vi "Billard2023.vi"() -> ()   [LabVIEW 2022 SP3]
doc: "This VI uses computer vision to score a game of french pool.\nSelect the sequence of png images you want to analyse and let the magic happen...\n\nAuthors : Romain Lattion & Ryan Svoboda"
panel:
  out "Running Matlab...":string
  out "percentage":dbl
  out "slide":dbl(slide) scale=0.0..100.0
  in  "Create Matlab scoresheet":bool
  in  "Line type":string(combo)="-*"
  in  "Band touch lose":u32(colorbox)=16711680
  in  "Band touch win":u32(colorbox)=65280
  in  "Select the sequence (folder)":path
  out "?":picture
  # "Romain Lattion & Ryan Svoboda"
  # "Billard 2023"
  # "Loading...       %"
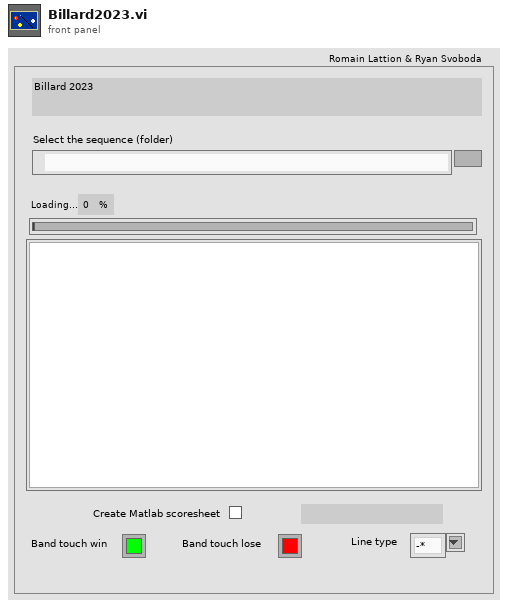
[diagram p1: front panel]
types:
  T1 = typedef "imagedata.ctl" = cluster{"image type":i32, "image depth":i32, "image":u8[], "mask":u8[], "colors":u32[], "Rectangle":cluster{"left":i16, "top":i16, "right":i16, "bottom":i16}}
  T2 = enum16{"open", "replace", "create", "open or create", "replace or create", "replace or create with confirmation"}
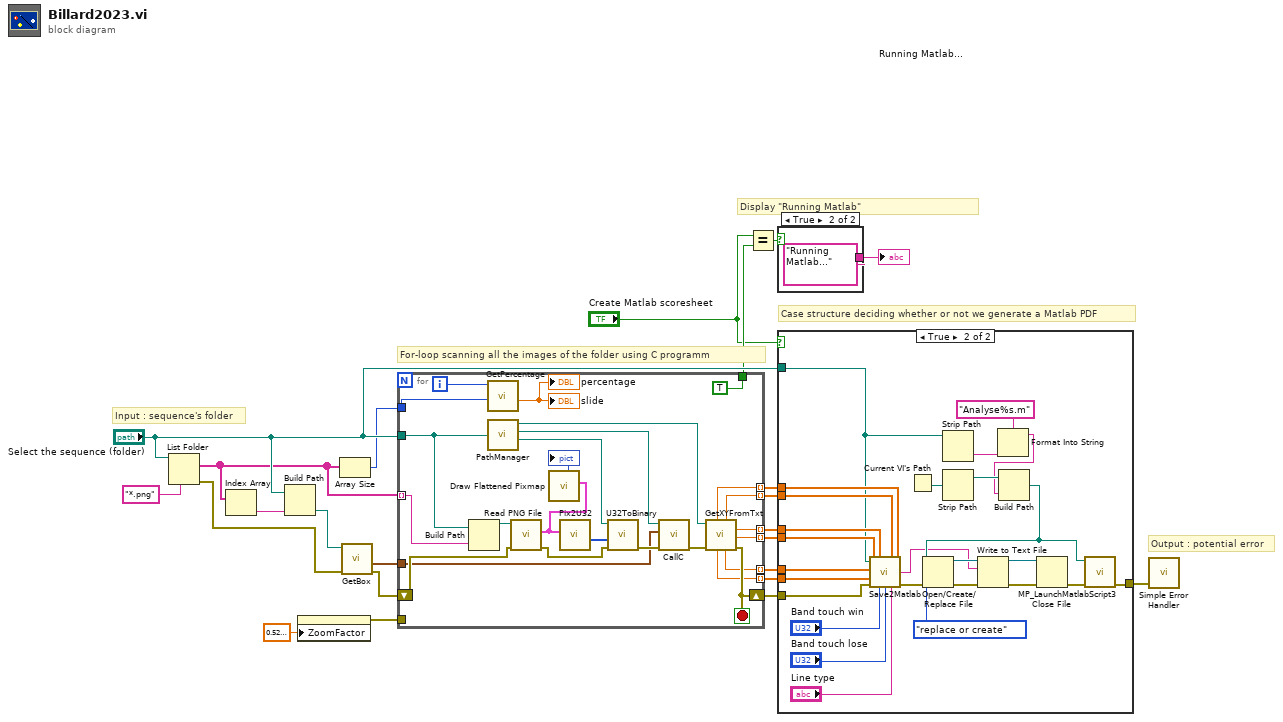
[diagram p0: block diagram]
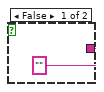
[diagram p2: hidden frame]
diagram:
  # "Output : potential error"
  # "Input : sequence's folder"
  # "Display \"Running Matlab\""
  # "Case structure deciding whether or not we generate a Matlab PDF"
  # "For-loop scanning all the images of the folder using C programm"
  n1 = List Folder(path="Select the sequence (folder)", pattern="*.png") -> (filenames=w12:string[], error out=w17:errorcluster)  [unwired: 2 in, 2 out]
  n2 = Index Array(array=w12) -> (element=w13:string)  [unwired: 1 in]
  n3 = Build Path(base path="Select the sequence (folder)", name or relative path=w13) -> (appended path=w18:path)
  n4 = property class="Pict"("ZoomFactor"=sgl 0.53 ("Zoom Factor")) -> (error out=w22:errorcluster)  [unwired: 2 in, 1 out]
  n5 = Array Size(array=w12) -> (size(s)=w11:i32)
  n6 = call "GetBox.vi"("error in (no error)"=w17, "path to a png image"=w18) -> ("error out"=w16:errorcluster, "edges coordinates"=w15:cluster{u32, u32, u32, u32})  [unwired: 8 in]
  n7 = for {
    tunnel: "Select the sequence (folder)" -> [w25]
    tunnel: w22 -> [_]
    shift-right: [w32] -> w20
    shift-left: w16 -> [w46]
    tunnel: [w26] -> w9 mode=indexing
    tunnel: [w28] -> w8 mode=indexing
    tunnel: [w31] -> w4 mode=indexing
    tunnel: [w30] -> w3 mode=indexing
    tunnel: [w29] -> w2 mode=indexing
    tunnel: [w27] -> w1 mode=indexing
    tunnel: w15 -> [w36]
    tunnel: w12 -> [w42] mode=indexing
    tunnel: w11 -> [w41]
    tunnel: [TRUE] -> w7
    i -> [w39]
    stop <- w32 stop-if-true
    n8 = Build Path(base path=w25, name or relative path=w42) -> (appended path=w48:path)
    n9 = call "GetPercentage.vi"("total number"=w41, "current number"=w39) -> ("percentage"=→"slide" →"percentage":dbl)  [unwired: 9 in]
    n10 = call "PathManager.vi"("path to sequence folder"=w25) -> ("path to Pixmap.bin"=w38:path, "path to Pix2Pos.exe"=w35:path, "path to Pos.txt"=w33:path)  [unwired: 8 in]
    n11 = call <vilib>:"Read PNG File.vi"("error in (no error)"=w46, "path to PNG file"=w48) -> ("error out"=w43:errorcluster, "image data"=w45:T1)  [unwired: 7 in, 1 out]
    n12 = call <vilib>:"Draw Flattened Pixmap.vi"("image data"=w45) -> ("new picture"=→"?":picture)  [unwired: 8 in]
    n13 = call "Pix2U32.vi"("input cluster"=w45) -> ("pixmap"=w44:u32[])  [unwired: 10 in]
    n14 = call "U32ToBinary.vi"("error in"=w43, "pixmap"=w44, "path to pixmap.bin"=w38) -> ("error out"=w37:errorcluster)  [unwired: 8 in]
    n15 = call "CallC.vi"("error in (no error)"=w37, "Edges"=w36, "path to Pix2Pos.exe"=w35) -> ("error out"=w34:errorcluster)  [unwired: 8 in]
    n16 = call "GetXYFromTxt.vi"("error in"=w34, "path to pos.txt"=w33) -> ("error out"=w32:errorcluster, "Yy"=w30:dbl, "Xy"=w31:dbl, "Xw"=w29:dbl, "Yr"=w28:dbl, "Yw"=w27:dbl, "Xr"=w26:dbl)  [unwired: 3 in]
  }
  n17 = Equal?(x="Create Matlab scoresheet", y=w7) -> (x = y?=w5:bool)
  n18 = case shown="True" w5 {
    tunnel: ["" "Running Matlab..."] -> w10
    frame False {
    }
    frame True {
    }
  }
  "Running Matlab..." <- w10
  n19 = case shown="True" "Create Matlab scoresheet" {
    tunnel: w20 -> [w51 w77]
    tunnel: [w51 w76] -> w19
    tunnel: "Select the sequence (folder)" -> [_ w52]
    tunnel: w9 -> [_ w75]
    tunnel: w8 -> [_ w74]
    tunnel: w4 -> [_ w73]
    tunnel: w3 -> [_ w72]
    tunnel: w2 -> [_ w71]
    tunnel: w1 -> [_ w70]
    frame False {
    }
    frame True {
      n20 = call "Save2Matlab.vi"("Xr"=w75, "Yr"=w74, "Line"="Line type", "Band touch loose"="Band touch lose", "Xy"=w73, "Band touch win"="Band touch win", "Yy"=w72, "Path"=w52, "Xw"=w71, "Yw"=w70, "error in (no error)"=w77) -> ("Completed Matlab script"=w53:string, "error out"=w56:errorcluster)  [unwired: 3 in]
      n21 = Current VI's Path() -> (path=w69:path)
      n22 = Strip Path(path=w52) -> (name=w62:string)  [unwired: 1 out]
      n23 = Strip Path(path=w69) -> (stripped path=w68:path)  [unwired: 1 out]
      n24 = Format Into String(format string="Analyse%s.m", w62) -> (resulting string=w61:string)  [unwired: 2 in, 1 out]
      n25 = Build Path(base path=w68, name or relative path=w61) -> (appended path=w58:path)
      n26 = Open/Create/Replace File(file path (use dialog)=w58, error in=w56, operation (0:open)=T2."replace or create") -> (refnum out=w67:refnum<file>, error out=w65:errorcluster)  [unwired: 3 in, 1 out]
      n27 = Write to Text File(file (use dialog)=w67, text=w53, error in=w65) -> (refnum out=w66:refnum<file>, error out=w64:errorcluster)  [unwired: 1 in, 1 out]
      n28 = Close File(refnum=w66, error in=w64) -> (error out=w59:errorcluster)  [unwired: 1 out]
      n29 = call "MP_LaunchMatlabScript3.vi"("error in (no error)"=w59, "matlab script with path"=w58) -> ("error out"=w76:errorcluster)  [unwired: 5 in, 4 out]
    }
  }
  n30 = call <vilib>:"Simple Error Handler.vi"("error in (no error)"=w19) -> ()  [unwired: 4 in, 5 out]
